vi "CTECalculator.vi"(1 "yp":dbl, 2 "xi":dbl, 3 "xp":dbl, 4 "yi1":dbl, 5 "xi1":dbl, 6 "yi":dbl) -> (0 "CTE":dbl)   [LabVIEW 2024]
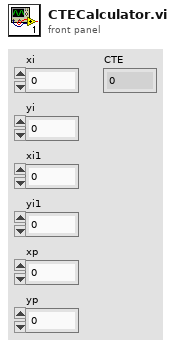
[diagram p1: front panel]
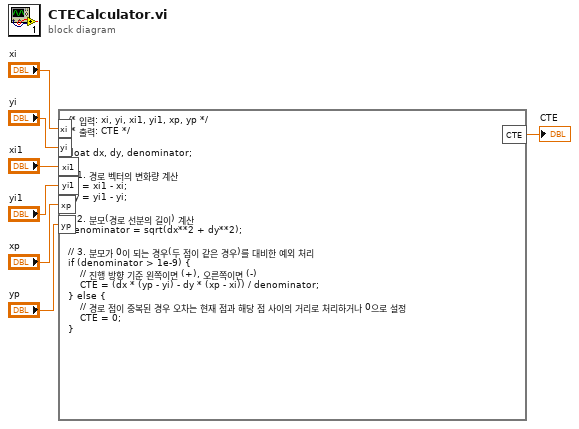
[diagram p0: block diagram]
diagram:
  n1 = formula code="/* 입력: xi, yi, xi1, yi1, xp, yp */\n/* 출력: CTE */\n\nfloat dx, dy, denominator;\n\n// 1. 경로 벡터의 변화량 계산\ndx = xi1 - xi;\ndy = yi1 - yi;\n\n// 2. 분모(경로 선분의 길이) 계산\ndenominator = sqrt(dx**2 + dy**2);\n\n// 3. 분모가 0이 되는 경우(두 점이 같은 경우)를 대비한 예외 처리\nif (denominator > 1e-9) {\n    // 진행 방향 기준 왼쪽이면 (+), 오른쪽이면 (-)\n    CTE = (dx * (yp - yi) - dy * (xp - xi)) / denominator;\n} else {\n    // 경로 점이 중복된 경우 오차는 현재 점과 해당 점 사이의 거리로 처리하거나 0으로 설정\n    CTE = 0; \n}"("xi"="xi", "yi"="yi", "xi1"="xi1", "yi1"="yi1", "xp"="xp", "yp"="yp") -> ("CTE"=→"CTE":dbl)
